vi "FlipArray.vi"() -> ()   [LabVIEW 2018]
panel:
  out "Array":i32[](array[numeric])
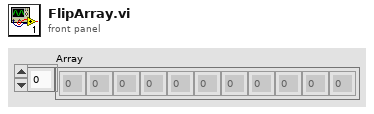
[diagram p1: front panel]
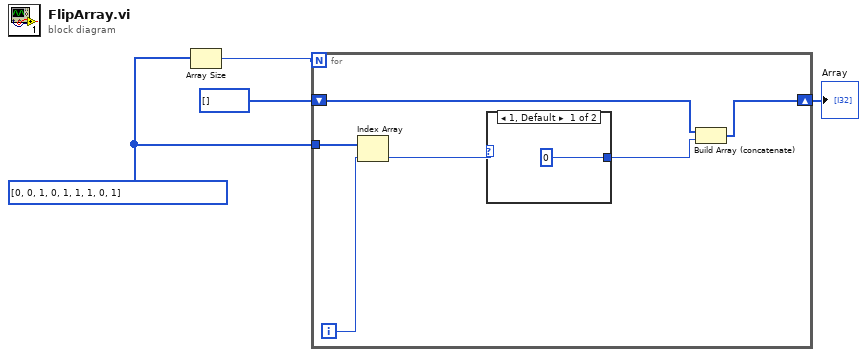
[diagram p0: block diagram]
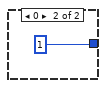
[diagram p2: hidden frame]
diagram:
  w3 = i32[] [0, 0, 1, 0, 1, 1, 1, 0, 1]
  n1 = Array Size(array=w3) -> (size(s)=w4:i32)
  n2 = for {
    N: w4 -> [_]
    tunnel: w3 -> [w10]
    shift-right: [w5] -> w1
    shift-left: i32[] [] -> [w6]
    i -> [w9]
    n3 = Index Array(array=w10, index=w9) -> (element=w8:i32)
    n4 = case shown="1, Default" w8 {
      tunnel: [0 1] -> w7
      frame 1, Default {
      }
      frame 0 {
      }
    }
    n5 = Build Array (concatenate)(w6, w7) -> (w5:i32[])
  }
  "Array" <- w1
